vi "LED Spike.vi"(8 "ON/OFF":bool, 11 "Mode":enum8{"Start", "Run", "Finish"}(ring)) -> ()   [LabVIEW 2014]
uses:
  <vilib>/Rock Robotics/WPI/Relay/WPI_RelayDirection.ctl
  <vilib>/Rock Robotics/SystemInterfaces/DIO/FPGA_DIORelayChannel.ctl
  <vilib>/Rock Robotics/WPI/Relay/WPI_RelayValue.ctl
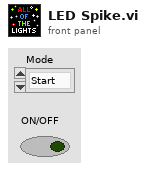
[diagram p1: front panel]
types:
  T1 = typedef "FPGA_DIORelayChannel.ctl" = enum8{"Relay 0", "Relay 1", "Relay 2", "Relay 3", "Invalid"}
  T2 = typedef "WPI_RelayDirection.ctl" = enum16{"Both directions", "Forward only", "Reverse only"}
  T3 = typedef "WPI_RelayValue.ctl" = enum16{"Off", "On", "Forward", "Reverse"}
  T4 = typedef "WPI_RelayDevRef.ctl" = cluster{"DevStatus":errorcluster, "Relay Channel":T1, "Controller":T5, "Relay Direction":T2}
  T5 = typedef "FPGA_TypedefDigitalModule.ctl" = enum16{"Controller 1"}
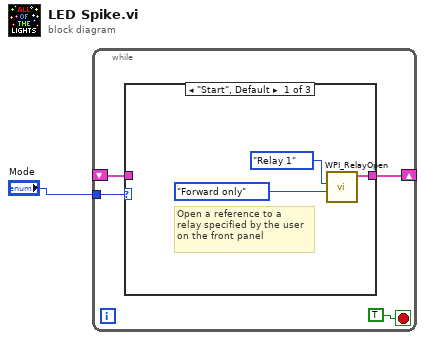
[diagram p0: block diagram]
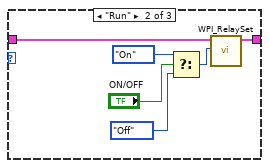
[diagram p2: hidden frame]
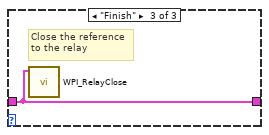
[diagram p3: hidden frame]
diagram:
  n1 = while {
    tunnel: "Mode" -> [w4]
    shift-right: [w3] -> _
    shift-left: _ -> [w2]
    stop <- TRUE stop-if-true
    n2 = case shown="\"Start\", Default" w4 {
      tunnel: [w6 w13 w15] -> w3
      tunnel: w2 -> [_ w14 w15]
      frame "Start", Default {
        # "Open a reference to a \nrelay specified by the user\non the front panel"
        n3 = call <vilib>:"WPI_RelayOpen.vi"("Relay Direction"=WPI_RelayDirection."Forward only" ("RelayDirection"), "Relay Channel"=FPGA_DIORelayChannel."Relay 1" ("RelayChannel")) -> ("RelayDevRef"=w6:T4)  [unwired: 2 in, 7 out]
      }
      frame "Run" {
        n4 = Select(t=WPI_RelayValue."On" ("RelayValue"), s="ON/OFF", f=WPI_RelayValue."Off" ("RelayValue")) -> (s? t:f=w10:T3)
        n5 = call <vilib>:"WPI_RelaySet.vi"("RelayValue"=w10, "RelayDevRef"=w14) -> ("RelayDevRef"=w13:T4)  [unwired: 1 in, 8 out]
      }
      frame "Finish" {
        # "Close the reference\nto the relay"
        n6 = call <vilib>:"WPI_RelayClose.vi"("RelayDevRef"=w15) -> ()  [unwired: 1 in, 10 out]
      }
    }
  }
